vi "Client Servo.vi"() -> ()   [LabVIEW 2015]
uses:
  <vilib>/MakerHub/LINX/Public/Sensors/Motion/Servo/Servo Open N Channels.vi
  <vilib>/MakerHub/LINX/Public/Sensors/Motion/Servo/Servo Set Pulse Width One Channel.vi
  <vilib>/MakerHub/LINX/Public/Sensors/Motion/Servo/Servo Close N Channels.vi
  <vilib>/MakerHub/LINX/LMH-LINX.lvlib
  <vilib>/MakerHub/LINX/Public/Sensors/Motion/Servo/Servo.lvlib
panel:
  in  "IO6":i8(knob) scale=-90.0..90.0
  in  "IO5":i8(knob) scale=-90.0..90.0
  in  "Connect":bool
  in  "About":bool
  in  "Stop":bool
  in  "VISA resource name":refnum<visa-resource-name>
  # "LabVIEW MakerHub"
  # "Proteus Test - Servo"
  # "COM Port"
  # "Servo 1"
  # "Servo 2"
  # "Quit"
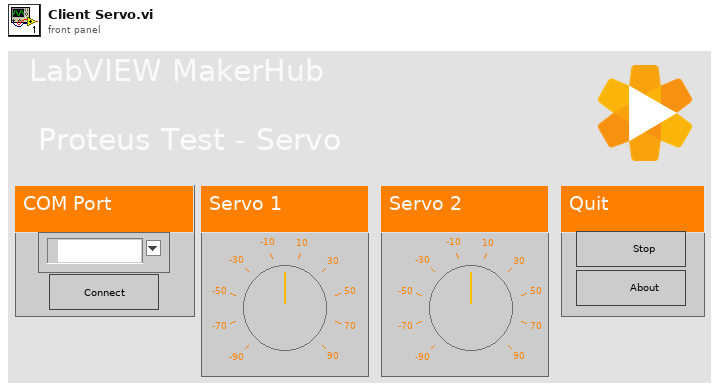
[diagram p1: front panel]
types:
  T1 = typedef "LMH-LINX.lvlib/LINX Ref.ctl" = cluster{"Platform":T2, "Interface":T3, "LINX Device Config":T4}
  T2 = typedef "LMH-LINX.lvlib/Platform.ctl" = enum16{"LINX", "myRIO"}
  T3 = typedef "LMH-LINX.lvlib/Interface.ctl" = enum16{"Serial", "TCP"}
  T4 = typedef "LMH-LINX.lvlib/Device.lvlib/LINX Device Config.ctl" = cluster{"Interface":T3, "COM Port":refnum<visa-resource-name>, "TCP Configuration":T5, "Device Family":u8, "Device ID":u8, "Device Name":string, "TCP Ref":refnum<k5>, "Channels":T6}
  T5 = typedef "LMH-LINX.lvlib/Device.lvlib/TCP Config.ctl" = cluster{"IP Address":string, "Port":u16}
  T6 = typedef "LMH-LINX.lvlib/Channels.ctl" = cluster{"DI":u8[], "DO":u8[], "AI":u8[], "AO":u8[], "PWM":u8[], "QE":u8[], "UART":u8[], "I2C 2":u8[], "SPI":u8[], "CAN":u8[], "Servo":u8[], "AI Ref (V)":dbl, "AO Ref (V)":dbl, "AO Resolution (Bits)":u8}
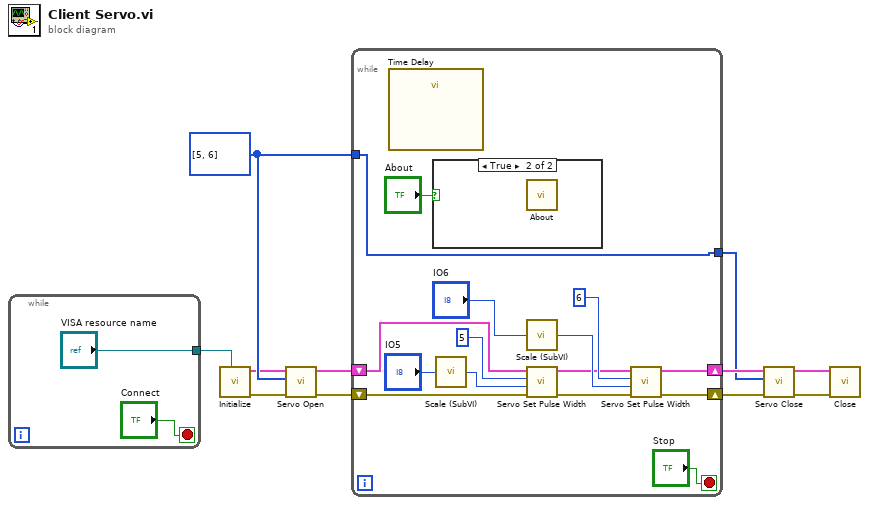
[diagram p0: block diagram]
diagram:
  w5 = u8[] [5, 6] ("Servo Channels")
  n1 = while {
    tunnel: ["VISA resource name"] -> w1
    stop <- "Connect" stop-if-true
  }
  n2 = call <vilib>:"Initialize.vi"("Serial Port"=w1) -> ("Error Out"=w2:errorcluster, "LINX Ref"=w3:T1)  [unwired: 8 in, 1 out]
  n3 = call-poly <vilib>:"Servo Open.vi"("Error In"=w2, "Servo Channels"=w5, "LINX Resource"=w3) -> ("Error Out"=w10:errorcluster, "LINX Resource"=w11:T1)  [unwired: 7 in]
  n4 = while {
    shift-right: [w15] -> w9
    shift-left: w11 -> [w26]
    shift-right: [w14] -> w8
    shift-left: w10 -> [w25]
    tunnel: w5 -> [w23]
    tunnel: [w23] -> w4
    stop <- "Stop" stop-if-true
    n5 = call "Time Delay"() -> ()  [unwired: 11 in, 1 out]
    n6 = case shown="True" "About" {
      frame False {
      }
      frame True {
        n7 = call "About.vi"() -> ()  [unwired: 1 in]
      }
    }
    n8 = call "Scale (SubVI).vi"("Desired Angle"="IO5") -> ("Servo Out"=w22:u16)
    n9 = call "Scale (SubVI).vi"("Desired Angle"="IO6") -> ("Servo Out"=w21:u16)
    n10 = call-poly <vilib>:"Servo Set Pulse Width.vi"("Error In"=w25, "Pulse Width (uS)"=w22, "Servo Channel"=u8 5, "LINX Resource"=w26) -> ("Error Out"=w18:errorcluster, "LINX Resource"=w19:T1)  [unwired: 6 in]
    n11 = call-poly <vilib>:"Servo Set Pulse Width.vi"("Error In"=w18, "Pulse Width (uS)"=w21, "Servo Channel"=u8 6, "LINX Resource"=w19) -> ("Error Out"=w14:errorcluster, "LINX Resource"=w15:T1)  [unwired: 6 in]
  }
  n12 = call-poly <vilib>:"Servo Close.vi"("Error In"=w8, "Servo Channels"=w4, "LINX Resource"=w9) -> ("Error Out"=w6:errorcluster, "LINX Resource"=w7:T1)  [unwired: 7 in]
  n13 = call <vilib>:"Close.vi"("Error In"=w6, "LINX Resource"=w7) -> ()  [unwired: 8 in, 2 out]
